vi "Create.vi"(7 "Direction":T1, 8 "error in (no error)":errorcluster, 9 "Custom Config Data":u8[](array[numeric]), 10 "Name":string, 11 "CIF_NIChn_FIFO_DAQ in":refnum<class "CIF_NIChn_FIFO_DAQ.lvclass">) -> (0 "error out":errorcluster, 3 "CIF_NIChn_FIFO_DAQ out":refnum<class "CIF_NIChn_FIFO_DAQ.lvclass">)   [LabVIEW 2021, in "CIF_NIChn_FIFO_DAQ.lvclass"]
uses:
  CIF_NIChn_FIFO_DAQ.lvclass
  D:/dev/Packages/Channel_Manager/src/CIFChannels/CIFChannels.lvclass
  D:/dev/Packages/Channel_Manager/src/CIF_NIChn/NIChn/CIF_NIChn.lvclass
  D:/dev/Packages/Channel_Manager/src/CIF_NIChn/FIFO_U8/CIF_NIChn_Fifo_U8.lvclass
  CIFChannels/Typedef/Direction.ctl
  <vilib>/CIF Foundation/CIF Utilities/Statistics/I64/Stats_I64_CIF_U.lvclass/Stats_I64_CIF_U.ctl
  CIFChannels/Typedef/Disconnect Behavior.ctl
  CIFChannels/CIFChannels.lvclass/CIFChannels.ctl
  ChannelCommon/typedef/Datatype Waveform.ctl
  CIFChannels/Typedef/Channel State.ctl
  CIF_NIChn_FIFO_DAQ.lvclass/CIF_NIChn_FIFO_DAQ.ctl
  NIChn/CIF_NIChn.lvclass/CIF_NIChn.ctl
  FIFO_U8/CIF_NIChn_Fifo_U8.lvclass/CIF_NIChn_Fifo_U8.ctl
  becc3daa-4a41-4263-a222-f735aa083fd2.vi
  7648bb3b-1ca8-489f-90cc-ebc9aace4b02.vi
  CIFChannels/Accessors/Write Channel State.vi
  NIChn/Accessors/Write CIF Channel.vi
  CIFChannels/Accessors/Write Channel Benchmark.vi
  CIFChannels/Accessors/Write Flatten Benchmark.vi
  FIFO_U8/Accessors/Write Payload.vi
  CIFChannels/SubVIs/Get Type from Class.vi
  ChannelCommon/Utilities/Unflatten FIFO Config.vi
  CIFChannels/Utilities/Apply Flags.vi
  CIFChannels/Accessors/Write Type.vi
  CIFChannels/Accessors/Write Channel Class.vi
  CIFChannels/Accessors/Write Direction.vi
  CIFChannels/Accessors/Write Tag Disconnect Behavior.vi
  CIFChannels/Accessors/Write Name.vi
  CIFChannels/Accessors/Write Custom Config Data.vi
  <vilib>/CIF Foundation/CIF Channels/CIFChannels/SubVIs/Add Error.vi
  becc3daa-4a41-4263-a222-f735aa083fd2.vi/c28b0ead-42ad-4072-80a2-aca7f2bd7ce3.vi
  <vilib>/CIF Foundation/CIF Channels/CIFChannels/SubVIs/CIFServices Fill In Error Info Ex.vi
  <vilib>/CIF Foundation/CIF Channels/CIFChannels/SubVIs/Get dll Path.vi
  becc3daa-4a41-4263-a222-f735aa083fd2.vi/259f1102-a6f3-45ef-83a9-e8a266e5a7b9.vi
  7648bb3b-1ca8-489f-90cc-ebc9aace4b02.vi/c28b0ead-42ad-4072-80a2-aca7f2bd7ce3.vi
  <vilib>/CIF Foundation/CIF Utilities/DataTypes/Unflatten U64.vi
  ChannelCommon/Utilities/Expand FIFO Flags.vi
  <vilib>/CIF Foundation/CIF Utilities/Errors/Append Error Location.vi
  <vilib>/Utility/LVClass/Get LV Class Name.vi
  <vilib>/CIF Foundation/CIF Utilities/Statistics/I64/Stats_I64_CIF_U.lvclass
  CIFChannels/CIFChannels.lvclass
  ChannelCommon/ChannelCommon.lvlib
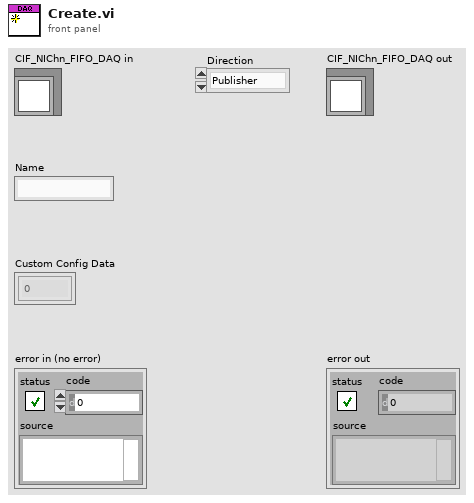
[diagram p1: front panel]
types:
  T1 = typedef "CIFChannels.lvclass/Direction.ctl" = enum16{"Publisher", "Subscriber"}
  T2 = typedef "CIFChannels.lvclass/Disconnect Behavior.ctl" = enum16{"Default value", "Last value", "Error with default"}
  T3 = typedef "ChannelCommon.lvlib/Datatype Waveform.ctl" = cluster{"measurement":dbl[], "dT":dbl, "Timestamp":i64, "Read Lock":bool}
  T4 = typedef "CIFChannels.lvclass/Channel State.ctl" = enum16{"Creating", "Disconnected", "Connecting", "Connected", "Destroyed"}
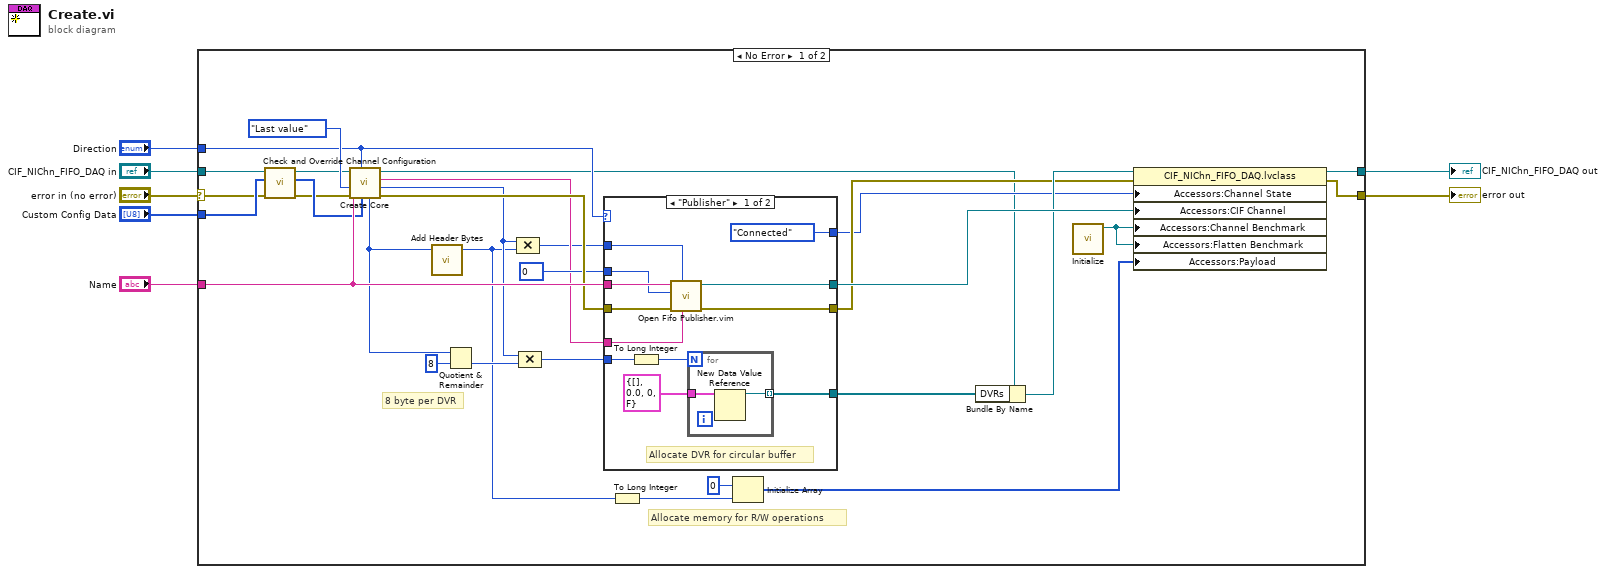
[diagram p0: block diagram]
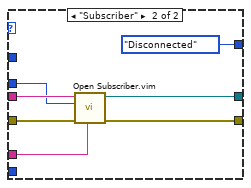
[diagram p2: hidden frame]
diagram:
  n1 = case shown="No Error" "error in (no error)" {
    selector: "error in (no error)" -> [w12 w61]
    tunnel: [w37 w61] -> w6
    tunnel: [w31 w60] -> w1
    tunnel: "CIF_NIChn_FIFO_DAQ in" -> [w15 w60]
    tunnel: "Name" -> [w36 _]
    tunnel: "Direction" -> [w30 _]
    tunnel: "Custom Config Data" -> [w14 _]
    frame No Error {
      # "8 byte per DVR"
      # "Allocate memory for R/W operations"
      n2 = call-dynamic "Check and Override Channel Configuration.vi"("error in (no error)"=w12, "Custom Config Data in"=w14, "CIF_NIChn_FIFO_DAQ in"=w15) -> ("error out"=w11:errorcluster, "Custom Config Data out"=w13:u8[], "CIF_NIChn_FIFO_DAQ out"=w10:refnum<class "CIF_NIChn_FIFO_DAQ.lvclass">)  [unwired: 6 in]
      n3 = call "Create Core.vi"("Custom Config Data"=w13, "Direction"=w30, "error in (no error)"=w11, "Disconnect Behavior"=Disconnect_Behavior."Last value", "Name"=w36, "CIFChannels in"=w10) -> ("error out"=w35:errorcluster, "Messages"=w18:u64, "Channel Type"=w27:string, "CIFChannels out"=w9:refnum<class "CIF_NIChn_FIFO_DAQ.lvclass">, "Bytes/Msg"=w17:u64)  [unwired: 1 in]
      n4 = call "Add Header Bytes.vi"("Bytes/Msg"=w17) -> ("Bytes/Msg with header"=w16:u64)  [unwired: 3 in]
      n5 = Quotient & Remainder(x=w17, y=u64 8) -> (floor(x/y)=w21:u64)  [unwired: 1 out]
      n6 = Compound Arithmetic op=MULTIPLY(w18, w16) -> (w25:u64)
      n7 = Compound Arithmetic op=MULTIPLY(w18, w21) -> (w20:u64)
      n8 = case shown="\"Publisher\"" w30 {
        tunnel: w36 -> [w50 w58]
        tunnel: w35 -> [w49 w57]
        tunnel: [w45 w53] -> w34
        tunnel: [w46 w54] -> w32
        tunnel: w27 -> [w48 w56]
        tunnel: [Channel_State."Connected" ("Channel State") Channel_State."Disconnected" ("Channel State")] -> w29
        tunnel: u8 0 -> [w44 w55]
        tunnel: w25 -> [w43 _]
        tunnel: w20 -> [w40 _]
        tunnel: [w42 _] -> w24
        frame "Publisher" {
          # "Allocate DVR for circular buffer"
          n9 = To Long Integer(number=w40) -> (32bit integer=w39:i32)
          n10 = call "Open Fifo Publisher.vim"("Channel Type Description"=w48, "depth"=w43, "error in"=w49, "Input Type"=w44, "Channel Name"=w50) -> ("error out"=w46:errorcluster, "CIF Channel"=w45:refnum<k21>)  [unwired: 5 in]
          n11 = for {
            N: w39 -> [_]
            tunnel: T3 {"measurement"=[], "dT"=0.0, "Timestamp"=0, "Read Lock"=FALSE} ("Waveform Datatype") -> [w52]
            tunnel: [w51] -> w42 mode=indexing
            n12 = New Data Value Reference(data value=w52) -> (data value reference=w51:refnum<data-value>)  [unwired: 1 in, 1 out]
          }
        }
        frame "Subscriber" {
          n13 = call "Open Subscriber.vim"("Channel Type Description"=w56, "error in"=w57, "Input Type"=w55, "Channel Name"=w58) -> ("error out"=w54:errorcluster, "CIF Channel"=w53:refnum<k21>)  [unwired: 6 in]
        }
      }
      n14 = To Long Integer(number=w16) -> (32bit integer=w19:i32)
      n15 = Initialize Array(u8 0 ("Numeric"), w19) -> (w8:u8[])
      n16 = Bundle By Name(cluster=w9, "DVRs"=w24) -> (w33:refnum<class "CIF_NIChn_FIFO_DAQ.lvclass">)
      n17 = call <vilib>:"Initialize.vi"() -> ("Stats_I64_CIF_U out"=w23:refnum<class "Stats_I64_CIF_U.lvclass">)  [unwired: 10 in, 1 out]
      n18 = property class="CIF_NIChn_FIFO_DAQ.lvclass"(reference=w33, error in=w32, "Accessors:Channel State"=w29, "Accessors:CIF Channel"=w34, "Accessors:Channel Benchmark"=w23, "Accessors:Flatten Benchmark"=w23, "Accessors:Payload"=w8) -> (reference out=w31:refnum<class "CIF_NIChn_FIFO_DAQ.lvclass">, error out=w37:errorcluster)
    }
    frame Error {
    }
  }
  "CIF_NIChn_FIFO_DAQ out" <- w1
  "error out" <- w6
